vi "Get Address Based Execution Time.vi"(8 "error in":errorcluster, 11 "timing section in":T1 format="%.0x") -> (0 "error out":errorcluster, 2 "address based execution time":T1 format="%.0x", 3 "timing section out":T1 format="%.0x")   [LabVIEW 2020, in "Ballard MIL-STD-1553 Scripting.lvlib"]
uses:
  Ballard MIL-STD-1553 Scripting.lvlib
  <vilib>/NI VeriStand/Custom Device API/Custom Device Item Ref.ctl
  Constants.vi
  <vilib>/NI VeriStand/Custom Device Tools/Custom Device Utility Library/Custom Device Utility Library.lvlib
  <vilib>/NI VeriStand/Custom Device API/Custom Device API.lvlib
  <vilib>/NI VeriStand/Custom Device Tools/Custom Device Utility Library/NI VeriStand - Search for Item by Name.vi
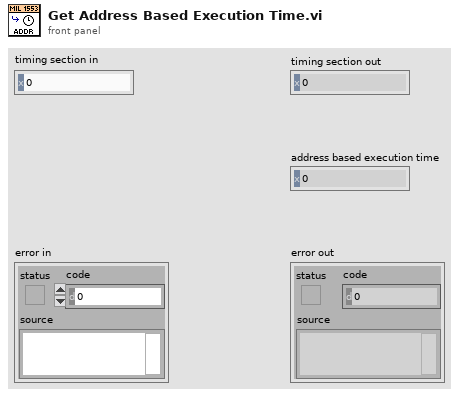
[diagram p1: front panel]
types:
  T1 = typedef "Custom Device API.lvlib/Custom Device Item Ref.ctl" = u64
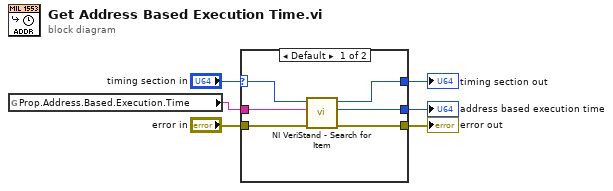
[diagram p0: block diagram]
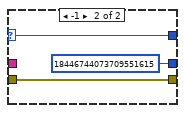
[diagram p2: hidden frame]
diagram:
  n1 = global read "Constants.vi" "Prop.Address.Based.Execution.Time"() -> (w1:string)
  n2 = case shown="Default" "timing section in" {
    selector: "timing section in" -> [w12 w15]
    tunnel: [w11 w14] -> w5
    tunnel: "error in" -> [w10 w14]
    tunnel: [w9 w15] -> w3
    tunnel: [w8 T1 18446744073709551615 ("Item Ref")] -> w2
    tunnel: w1 -> [w7 _]
    frame Default {
      n3 = call-poly <vilib>:"NI VeriStand - Search for Item.vi"("error in"=w10, "Item Name"=w7, "Section Ref in"=w12) -> ("error out"=w11:errorcluster, "Item Ref"=w8:T1, "Section Ref out"=w9:T1)  [unwired: 5 in, 1 out]
    }
    frame -1 {
    }
  }
  "error out" <- w5
  "timing section out" <- w3
  "address based execution time" <- w2
